vi "Validate Checksum.vi"(7 "Message In":T1, 11 "Error In":errorcluster) -> (8 "Message Out":T1, 10 "Valid?":bool, 15 "Error Out":errorcluster)   [LabVIEW 2023, in "ICanCommunicate.lvclass"]
doc: "Recalculates checksum for message and compares it with attached cheksum."
uses:
  ICanCommunicate.lvclass
  Message.ctl
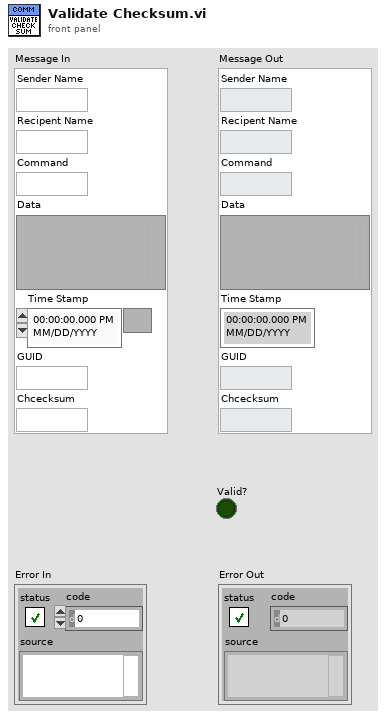
[diagram p1: front panel]
types:
  T1 = typedef "ICanCommunicate.lvclass/Message.ctl" = cluster{"Sender Name":string, "Recipent Name":string, "Command":string, "Data":variant, "Time Stamp":timestamp, "GUID":string, "Chcecksum":string}
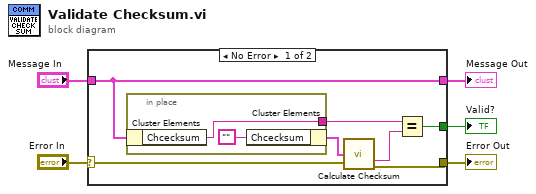
[diagram p0: block diagram]
diagram:
  n1 = case shown="No Error" "Error In" {
    selector: "Error In" -> [w11 w16]
    tunnel: [w9 w16] -> w4
    tunnel: "Message In" -> [w7 w15]
    tunnel: [w7 w15] -> w2
    tunnel: [w10 _] -> w1
    frame No Error {
      n2 = in-place {
        in-place-border: [w13] -> w8
        n3 = in-place-cluster #1(w7) -> ("Chcecksum"=w13:string)
        n4 = in-place-cluster #1("Chcecksum"="") -> (w6:T1)
      }
      n5 = call "Calculate Checksum.vi"("Message In"=w6, "Error In"=w11) -> ("Checksum"=w12:string, "Error Out"=w9:errorcluster)  [unwired: 11 in, 1 out]
      n6 = Equal?(x=w8, y=w12) -> (x = y?=w10:bool)
    }
    frame Error {
    }
  }
  "Error Out" <- w4
  "Message Out" <- w2
  "Valid?" <- w1
